vi "tcs_logEvent_wfpDataReady.vi"(8 "error in (no error)":errorcluster, 11 "logevent_wfpDataReady_Ctl":T1) -> (0 "error out":errorcluster, 2 "function return":i32, 3 "logevent_wfpDataReady_Ctl out":T1)   [LabVIEW 2016, in "SALLV_tcs.lvlib"]
doc: "int tcs_shm_logEvent_wfpDataReadyLV(tcs_logevent_wfpDataReadyLV *logevent_wfpDataReady_Ctl );"
uses:
  SALLV_tcs.lvlib
  DataTypes/logevent_wfpDataReady.ctl
  SALLV_tcs.so
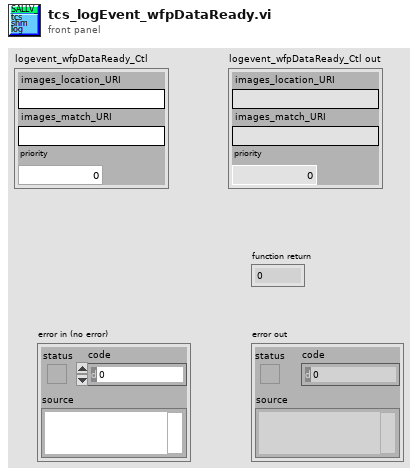
[diagram p1: front panel]
types:
  T1 = typedef "SALLV_tcs.lvlib/logevent_wfpDataReady.ctl" = cluster{"images_location_URI":string, "images_match_URI":string, "priority":i32}
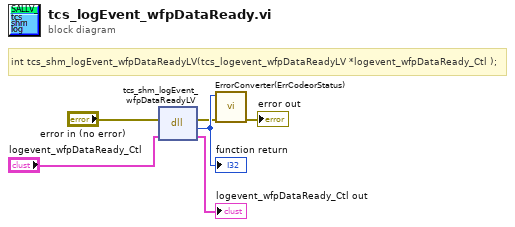
[diagram p0: block diagram]
diagram:
  # "int tcs_shm_logEvent_wfpDataReadyLV(tcs_logevent_wfpDataReadyLV *logevent_wfpDataReady_Ctl );"
  n1 = dll-call lib="home/andres/Desktop/SALLV_tcs/SALLV_tcs.*" fn="tcs_shm_logEvent_wfpDataReadyLV"(error in="error in (no error)", "logevent_wfpDataReady_Ctl"="logevent_wfpDataReady_Ctl") -> (error out=w2:errorcluster, w6:i32, "logevent_wfpDataReady_Ctl"=→"logevent_wfpDataReady_Ctl out":T1)  [unwired: 2 in, 1 out]
  "function return" <- w6
  n2 = call "ErrorConverter(ErrCodeorStatus).vi"("error in (no error)"=w2, "error code"=w6) -> ("error out"=→"error out":errorcluster)  [unwired: 9 in]
